vi "Initialize Threads.vi"(5 "FIFO Options":T1, 6 "Logging Interface":refnum<class "Logging Interface.lvclass">, 7 "Plugin Configuration":refnum<class "Plugin Configuration.lvclass">, 8 "error in (no error)":errorcluster, 9 "Components":refnum<class "Component.lvclass">[](array[class]), 10 "Transfer Groups":refnum<class "Transfer Group.lvclass">[](array[class]), 11 "Plugin in":refnum<class "Plugin.lvclass">) -> (0 "error out":errorcluster, 2 "Plugin Threads":refnum<class "Plugin Thread.lvclass">[](array[class]), 3 "Plugin out":refnum<class "Plugin.lvclass">)   [LabVIEW 2017, in "DSF Core.lvlib" / "Plugin.lvclass"]
uses:
  Plugin.lvclass
  Component/Component.lvclass
  Configuration/Core/Plugin/Plugin Configuration.lvclass
  Typedefs/DSF FIFO Options.ctl
  Thread/Plugin/Plugin Thread.lvclass
  Transfer Group/Transfer Group.lvclass
  Interface/Logging/Logging Interface.lvclass
  Thread/Plugin/Transceiver/Transceiver Thread.lvclass
  C:/Git/DSF/Core/Classes/Thread/Plugin/Plugin Thread.lvclass
  Configuration/Core/Plugin/Plugin Configuration.lvclass/Plugin Configuration.ctl
  Plugin.lvclass/Plugin.ctl
  Configuration/Core/Thread/Thread Configuration.lvclass
  Framework/Framework.lvclass
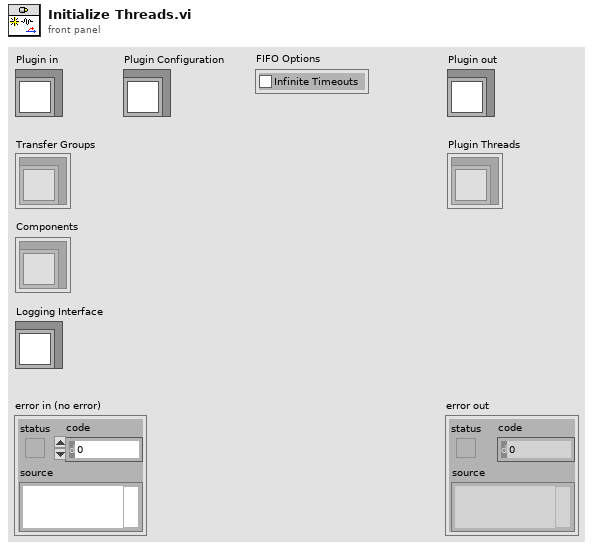
[diagram p1: front panel]
types:
  T1 = typedef "DSF Core.lvlib/Framework.lvclass/DSF FIFO Options.ctl" = cluster{"Infinite Timeouts":bool}
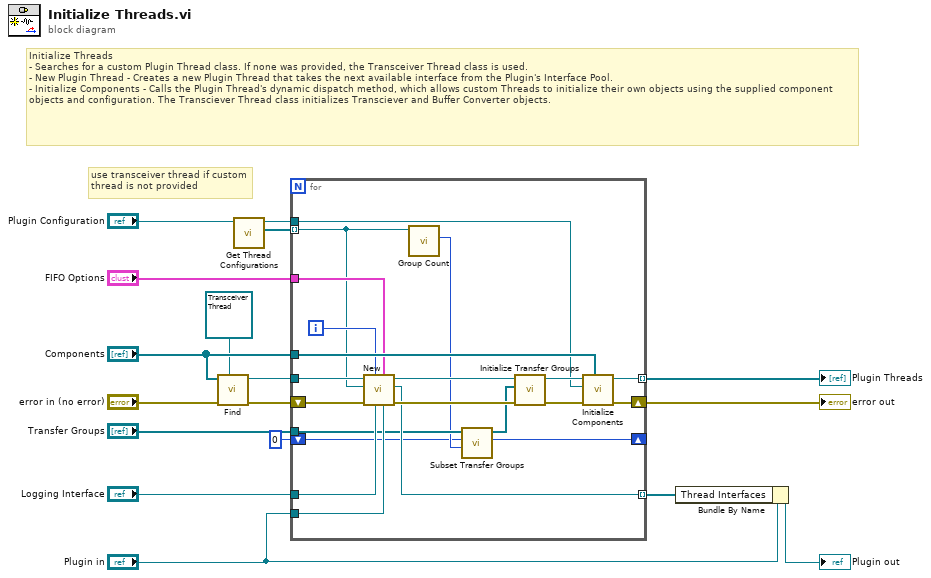
[diagram p0: block diagram]
diagram:
  # "Initialize Threads\n- Searches for a custom Plugin Thread class. If none was provided, the Transceiver Thread class is used.\n- New Plugin Thread - Creates a new Plugin Thread that takes the next available interface from the Plugin's Interface Pool.\n- Initialize Components - Calls the Plugin Thread's dynamic dispatch method, which allows custom Threads to initialize their own objects using the supplied component objects and configuration. The Transciever Thread class initializes Transciever and Buffer Converter objects."
  # "use transceiver thread if custom thread is not provided"
  n1 = call "Find.vi"("default"=refnum<class "Transceiver Thread.lvclass"> refnum ("DSF Core.lvlib:Transceiver Thread.lvclass"), "error in (no error)"="error in (no error)", "Components"="Components") -> ("error out"=w12:errorcluster, "Plugin Thread"=w8:refnum<class "Plugin Thread.lvclass">)  [unwired: 6 in, 1 out]
  n2 = call "Get Thread Configurations.vi"("Plugin Configuration in"="Plugin Configuration") -> ("Thread Configurations"=w3:refnum<class "Thread Configuration.lvclass">[], "Plugin Configuration out"=w1:refnum<class "Plugin Configuration.lvclass">)  [unwired: 8 in, 1 out]
  n3 = for {
    shift-right: [w37] -> w16
    shift-left: w12 -> [w32]
    tunnel: "Transfer Groups" -> [w24]
    tunnel: [w38] -> w17 mode=indexing
    tunnel: w3 -> [w23] mode=indexing
    tunnel: "Components" -> [w36]
    tunnel: w8 -> [w31]
    tunnel: "Logging Interface" -> [w35]
    tunnel: "Plugin in" -> [w34]
    tunnel: "FIFO Options" -> [w33]
    tunnel: [w27] -> w9 mode=indexing
    shift-right: [w21] -> _
    shift-left: 0 ("index + count") -> [w20]
    tunnel: w1 -> [w18]
    i -> [w26]
    n4 = call "New.vi"("Plugin"=w34, "FIFO Options"=w33, "Logging Interface"=w35, "thread ID"=w26, "error in (no error)"=w32, "Thread Configuration"=w23, "Plugin Thread type"=w31) -> ("error out"=w30:errorcluster, "Plugin Thread Interface"=w27:refnum<class "Plugin Interface.lvclass">, "Plugin Thread out"=w29:refnum<class "Plugin Thread.lvclass">)  [unwired: 2 in]
    n5 = call-dynamic "Group Count.vi"("Thread Configuration in"=w23) -> ("group count"=w22:i32)  [unwired: 8 in, 2 out]
    n6 = call "Subset Transfer Groups.vi"("count"=w22, "index"=w20, "Transfer Groups"=w24) -> ("index + count"=w21:i32, "subset Transfer Groups"=w19:refnum<class "Transfer Group.lvclass">[])  [unwired: 6 in, 1 out]
    n7 = call "Initialize Transfer Groups.vi"("error in (no error)"=w30, "Transfer Groups"=w19, "Plugin Thread in"=w29) -> ("error out"=w25:errorcluster, "Plugin Thread out"=w28:refnum<class "Plugin Thread.lvclass">)  [unwired: 7 in]
    n8 = call-dynamic "Initialize Components.vi"("Components"=w36, "error in (no error)"=w25, "Plugin Configuration"=w18, "Plugin Thread in"=w28) -> ("error out"=w37:errorcluster, "Plugin Thread out"=w38:refnum<class "Plugin Thread.lvclass">)  [unwired: 6 in]
  }
  "error out" <- w16
  "Plugin Threads" <- w17
  n9 = Bundle By Name(cluster="Plugin in", "Thread Interfaces"=w9) -> (→"Plugin out":refnum<class "Plugin.lvclass">)
